vi "signal_generate.vi"(8 "error in":errorcluster, 9 "sampling info":cluster{"Fs":dbl, "#s":dbl}={"Fs"=100000000.0, "#s"=100000.0} {"Fs" format="%.2p"}, 11 "module path":path) -> (0 "error out":errorcluster, 2 "Predicted params":T1)   [LabVIEW 2023]
uses:
  <vilib>/numeric/Random Number (Range) DBL.vi
  <vilib>/measure/NI_MABase.lvlib
panel:
  in  "stop":bool
  in  "Predict":bool
  in  "Noise":bool
  in  "Signal":bool
  out "Waveform Graph":waveform(dbl)(graph)
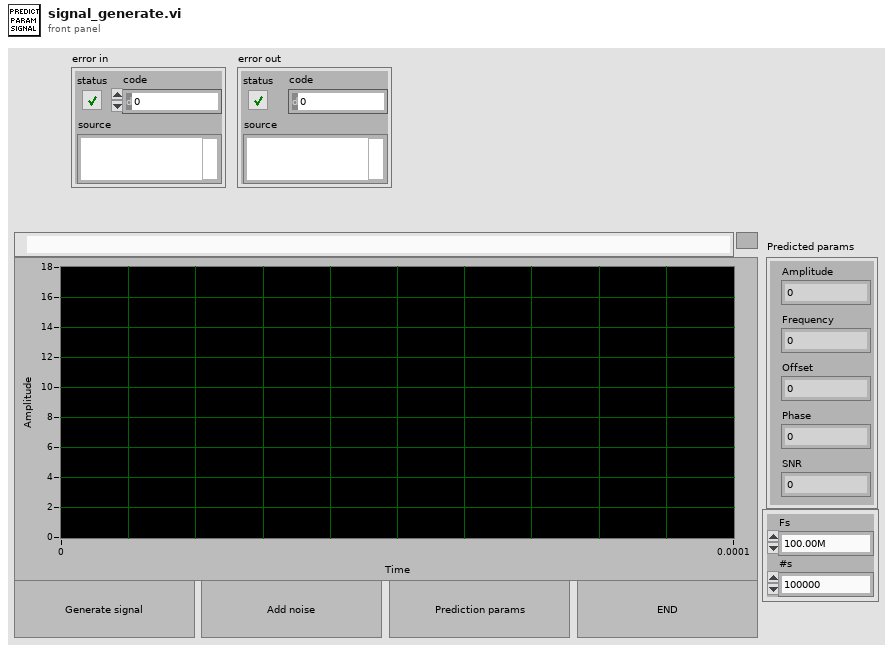
[diagram p1: front panel]
types:
  T1 = cluster{"Amplitude":dbl, "Frequency":dbl, "Offset":dbl, "Phase":dbl, "SNR":dbl}
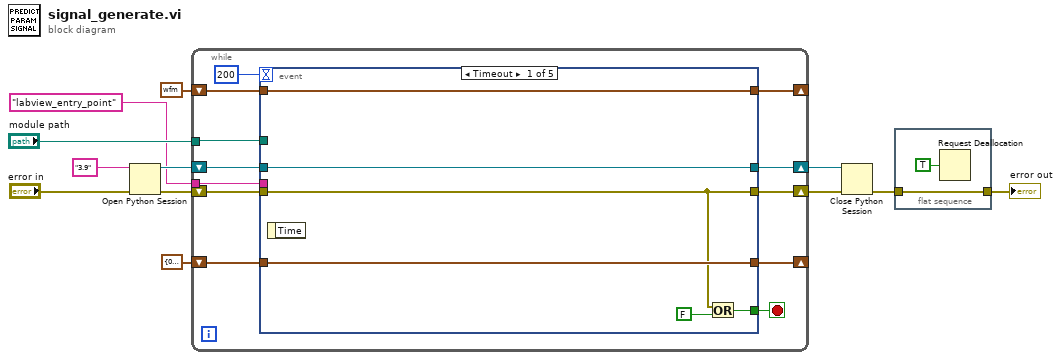
[diagram p0: block diagram]
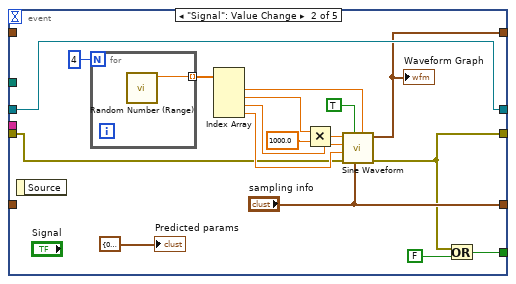
[diagram p2: hidden frame]
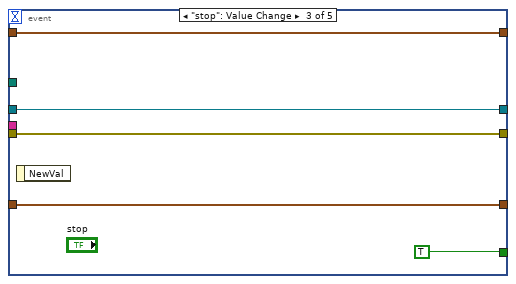
[diagram p3: hidden frame]
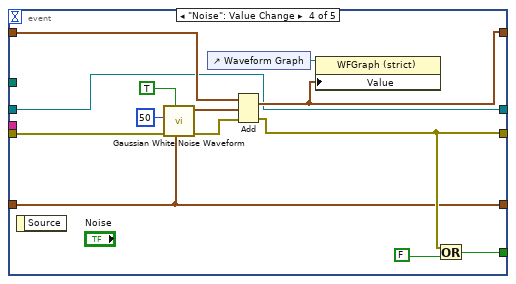
[diagram p4: hidden frame]
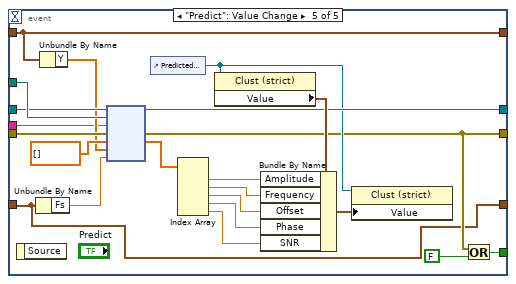
[diagram p5: hidden frame]
diagram:
  n1 = Open Python Session(python version="3.9" ("Python version"), 3:"error in") -> (session out=w8:refnum<k35>, error out=w9:errorcluster)  [unwired: 1 in]
  n2 = while {
    tunnel: "module path" -> [w22]
    shift-right: [w19] -> w6
    shift-left: w8 -> [w20]
    shift-right: [w18] -> w7
    shift-left: w9 -> [w21]
    shift-right: [w16] -> _
    shift-left: cluster{"Fs":dbl, "#s":dbl} {"Fs"=0.0, "#s"=0.0} ("sampling info") -> [w17]
    shift-right: [w15] -> _
    shift-left: waveform(dbl) {"t0"=timestamp(0 s since 1904-01-01), "dt"=1.0, "Y"=[]} ("signal out") -> [w14]
    tunnel: "labview_entry_point" ("function name") -> [w13]
    stop <- w23 stop-if-true
    n3 = event shown="[0] Timeout" {
      selector: _ -> [_ _ _ _ _]
      dyn-events: _ -> [_ _ _ _ _]
      timeout: 200 -> [_ _ _ _ _]
      tunnel: [w27 w33 TRUE w59 w73] -> w23
      tunnel: w22 -> [_ _ _ _ w88]
      tunnel: w21 -> [w26 w37 w50 w65 w87]
      tunnel: w20 -> [w29 w35 w52 w56 w86]
      tunnel: [w29 w35 w52 w56 w77] -> w19
      tunnel: [w26 w31 w50 w58 w72] -> w18
      tunnel: w17 -> [w30 _ w53 w55 w67]
      tunnel: [w30 "sampling info" w53 w55 w67] -> w16
      tunnel: [w28 w34 w51 w60 w69] -> w15
      tunnel: w14 -> [w28 _ w51 w63 w69]
      tunnel: w13 -> [_ _ _ _ w68]
      event Timeout {
        n4 = event-data() -> ()  [unwired: 1 in, 1 out]
        n5 = Or(x=w26, y=FALSE) -> (x .or. y?=w27:bool)
      }
      event "Signal": Value Change {
        n6 = event-data() -> ()  [unwired: 1 in, 1 out]
        n7 = for {
          N: 4 -> [_]
          tunnel: [w48] -> w44 mode=indexing
          n8 = call-poly <vilib>:"Random Number (Range).vi"() -> ("number"=w48:dbl)  [unwired: 11 in]
        }
        n9 = Index Array(array=w44) -> (element #1=w43:dbl, element #2=w41:dbl, element #3=w39:dbl, element #4=w38:dbl)  [unwired: 4 in]
        n10 = Multiply(x=w41, y=1000.0) -> (x*y=w42:dbl)
        n11 = call <vilib>:"Sine Waveform.vi"("offset"=w43, "sampling info"="sampling info", "reset signal"=TRUE, "error in (no error)"=w37, "phase"=w38, "amplitude"=w39, "frequency"=w42) -> ("error out"=w31:errorcluster, "signal out"=w34:waveform(dbl))  [unwired: 3 in]
        "Waveform Graph" <- w34
        n12 = Or(x=w31, y=FALSE) -> (x .or. y?=w33:bool)
        "Predicted params" <- T1 {"Amplitude"=0.0, "Frequency"=0.0, "Offset"=0.0, "Phase"=0.0, "SNR"=0.0} ("Predicted params")
      }
      event "stop": Value Change {
        n13 = event-data() -> ()  [unwired: 1 in, 1 out]
      }
      event "Noise": Value Change {
        n14 = event-data() -> ()  [unwired: 1 in, 1 out]
        n15 = call <vilib>:"Gaussian White Noise Waveform.vi"("sampling info"=w55, "reset signal"=TRUE, "error in (no error)"=w65, "seed"=50) -> ("error out"=w62:errorcluster, "signal out"=w64:waveform(dbl))  [unwired: 6 in]
        n16 = control-ref of="Waveform Graph"() -> (w61:refnum<vi>)
        n17 = Add(1:w64, 2:w63, 4:w62) -> (0:w60:waveform(dbl), 3:w58:errorcluster)
        n18 = property class="WFGraph (strict)"(reference=w61, "Value"=w60) -> ()  [unwired: 1 in, 2 out]
        n19 = Or(x=w58, y=FALSE) -> (x .or. y?=w59:bool)
      }
      event "Predict": Value Change {
        n20 = event-data() -> ()  [unwired: 1 in, 1 out]
        n21 = Unbundle By Name(w67) -> ("Fs"=w71:dbl)
        n22 = Unbundle By Name(w69) -> ("Y"=w70:dbl[])
        n23 = node(w86, w88, w68, w87, dbl[] [], w70, w71) -> (w77:refnum<k35>, w72:errorcluster, w80:dbl[])  [unwired: 2 in, 2 out]
        n24 = control-ref of="Predicted params"() -> (w75:refnum<vi>)
        n25 = Index Array(array=w80) -> (element #1=w81:dbl, element #2=w82:dbl, element #3=w85:dbl, element #4=w83:dbl, element #5=w84:dbl)  [unwired: 5 in]
        n26 = property class="Clust (strict)"(reference=w75) -> ("Value"=w78:T1)  [unwired: 1 in, 2 out]
        n27 = Bundle By Name(cluster=w78, "Amplitude"=w81, "Frequency"=w82, "Offset"=w85, "Phase"=w83, "SNR"=w84) -> (w76:T1)
        n28 = property class="Clust (strict)"(reference=w75, "Value"=w76) -> ()  [unwired: 1 in, 2 out]
        n29 = Or(x=w72, y=FALSE) -> (x .or. y?=w73:bool)
      }
    }
  }
  n30 = Close Python Session(session in=w6, error in=w7) -> (11:w2:errorcluster)
  n31 = flat-sequence {
    tunnel: w2 -> [w90]
    tunnel: [w90] -> w1
    frame #0 {
      n32 = Request Deallocation(TRUE ("flag")) -> ()
    }
  }
  "error out" <- w1
